vi "OPCUA AddTagToGroup.vi"(8 "error in (no error)":errorcluster, 9 "Tag":string, 10 "SamplingInterval":i32=250, 11 "reference":refnum<k24>) -> (0 "error out":errorcluster, 3 "reference 2":refnum<k24>)   [LabVIEW 2019]
uses:
  F:/src/HUTCDLSVN/Machine/CDL0100/TagEngine/LVOPCUA.NET/LVOPC.NETInterface/bin/Release/LVOPC.NETInterface.dll
  LVOPCUA.NET/LVOPC.NETInterface/bin/Release/LVOPC.NETInterface.dll
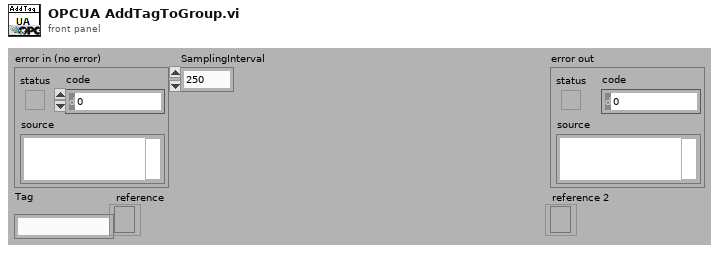
[diagram p1: front panel]
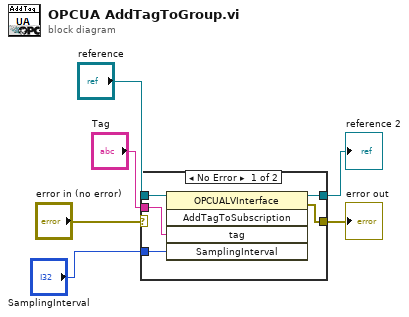
[diagram p0: block diagram]
diagram:
  n1 = case shown="No Error" "error in (no error)" {
    selector: "error in (no error)" -> [_ w13]
    tunnel: "Tag" -> [w10 _]
    tunnel: [w9 w13] -> w5
    tunnel: "reference" -> [w11 w12]
    tunnel: [w8 w12] -> w2
    tunnel: "SamplingInterval" -> [w7 _]
    frame No Error {
      n2 = invoke class="OPCUALVInterface" method="AddTagToSubscription"(reference=w11, "tag"=w10, "SamplingInterval"=w7) -> (reference out=w8:refnum<k24>, error out=w9:errorcluster)  [unwired: 2 in, 3 out]
    }
    frame Error {
    }
  }
  "error out" <- w5
  "reference 2" <- w2
